vi "Main.vi"() -> ()   [LabVIEW 2017]
doc: "The myRIO Project template acquires acceleration data from the onboard accelerometer and displays the changes of acceleration values in a waveform chart."
uses:
  Motor Status Enum.ctl
  Motion Type Def.ctl
  XY Cluster.ctl
  <vilib>/addons/control/pid/pid.llb/PID Control Input Filter (DBL).vi
  <vilib>/addons/control/pid/pid.llb/PID (DBL).vi
  <vilib>/addons/control/pid/NI_PID_pid.lvlib
  <vilib>/ptbypt/NI_PtbyPt.lvlib
panel:
  out "Y Data.Path.Decel Dist":dbl
  out "X Data.Path.Decel Dist":dbl
  out "Y dist > +20":bool
  out "X dist > +20":bool
  out "Y Data.Path. Profile":T1=enum."Triangular"
  out "X Data.Path.Profile":T1=enum."Triangular"
  out "Timing":T2
  out "Y V Array":dbl[](array[numeric])
  out "X V Array":dbl[](array[numeric])
  out "Y PID":cluster{"Speed":dbl, "Speed":dbl}(graph)
  out "X PID":cluster{"Speed":dbl, "Speed":dbl}(graph)
  out "Y Data.State":T3
  out "X Data.State":T3
  out "X PID Output":dbl format="%.2f"
  out "Y PID Output":dbl format="%.2f"
  in  "Y Input":T4
  in  "Y Axis PID":cluster{"Kc":dbl, "Ti":dbl, "Td":dbl}
  in  "X Input":T4
  in  "X Axis PID":cluster{"Kc":dbl, "Ti":dbl, "Td":dbl}
  in  "stop":bool
  out "X&Y Complete":bool
  out "Y Freq":dbl(graph)
  out "X Duty%":dbl(graph)
  out "Y Acceleration":dbl[](graph)
  out "Y Displacement":dbl[](graph)
  out "X Acceleration":dbl[](graph)
  out "X Displacement":dbl[](graph)
  out "Y Velocity":cluster{"V actual":dbl[]}[](graph)
  out "X Velocity":cluster{"V actual":dbl[]}[](graph)
  out "Y Data.Motion":T5
  out "X Data.Motion":T5
  out "Y Data.Motor Params":T6
  out "X Data.Motor Params":T7
  # "X MaxV = 26.73 mm/s at 50 Hz"
  # "Y MaxV = 14.38 mm/s at 3200 µSteps/rev"
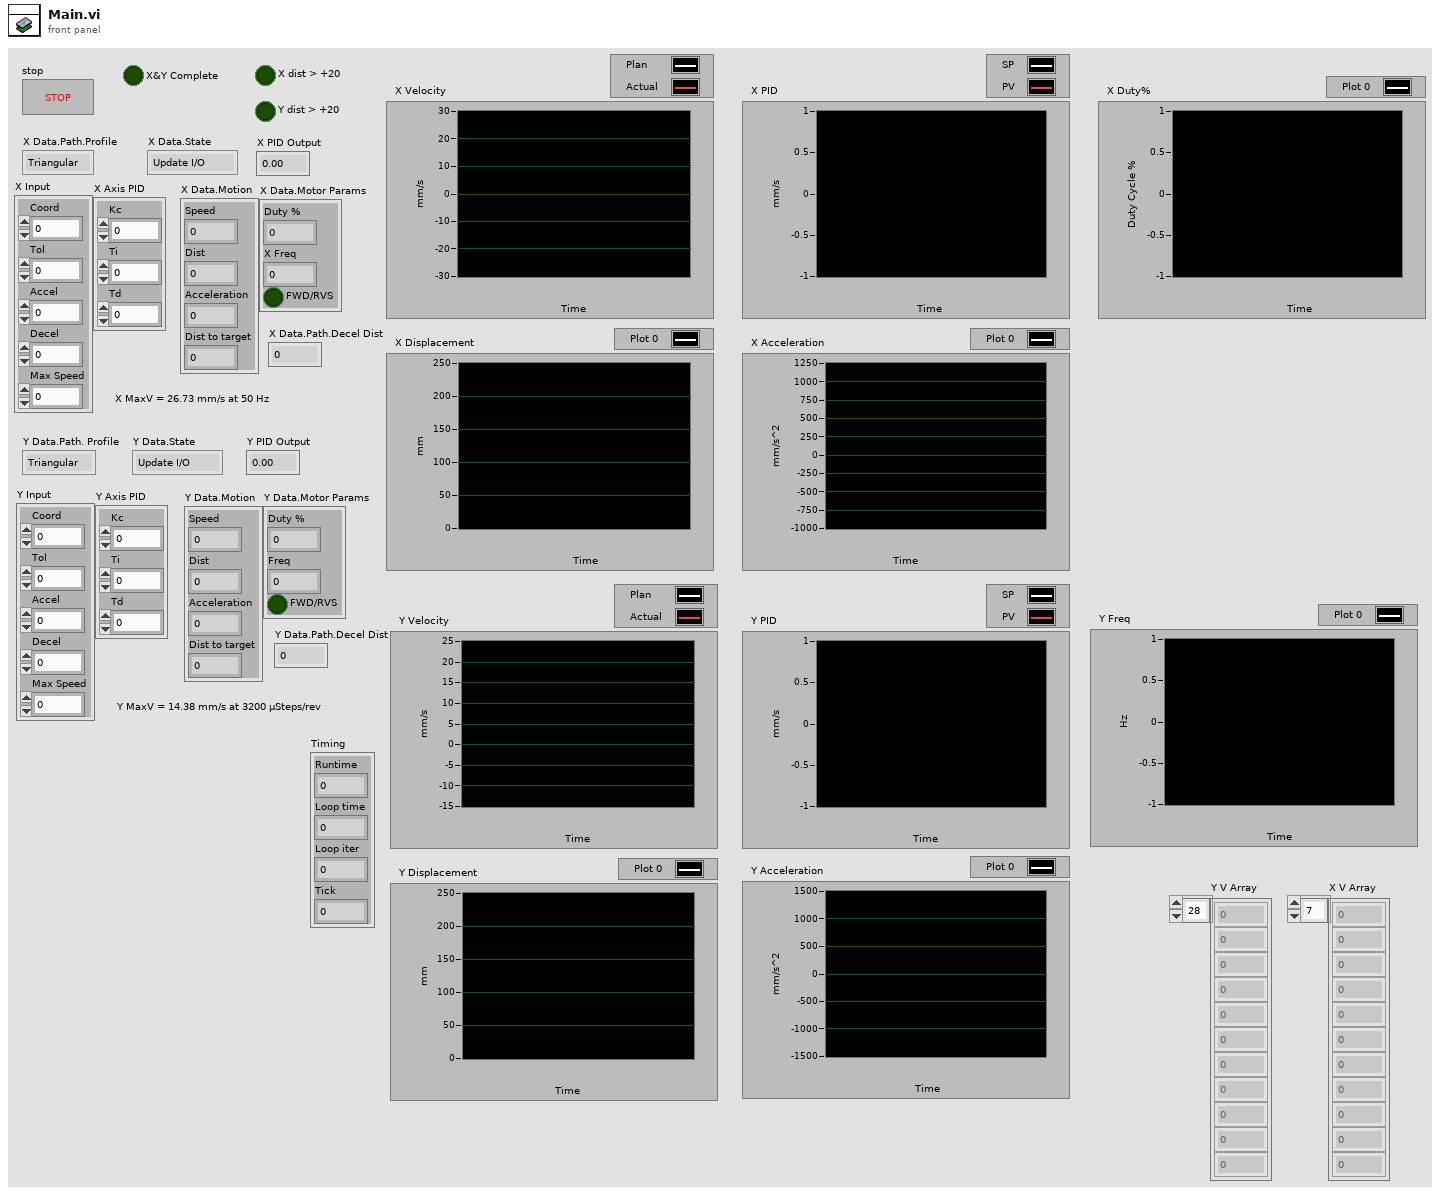
[diagram p1: front panel]
types:
  T1 = typedef "Motion Type Def.ctl" = enum16{"Trapezodial", "Triangular"}
  T2 = cluster{"Runtime":dbl, "Loop time":dbl, "Loop iter":i32, "Tick":dbl}
  T3 = typedef "Motor Status Enum.ctl" = enum16{"Update I/O", "Stop", "Steady Speed", "Accelerate", "Decelerate", "Drive Motor"}
  T4 = cluster{"Coord":dbl, "Tol":dbl, "Accel":dbl, "Decel":dbl, "Max Speed":dbl}
  T5 = cluster{"Speed":dbl, "Dist":dbl, "Acceleration":dbl, "Dist to target":dbl}
  T6 = cluster{"Duty %":dbl, "Freq":dbl, "FWD/RVS":bool}
  T7 = cluster{"Duty %":dbl, "X Freq":dbl, "FWD/RVS":bool}
  T8 = typedef "XY Cluster.ctl" = cluster{"X Data":cluster{"Complete?":bool, "Motor Params":cluster{"Duty %":dbl, "X Freq":dbl, "FWD/RVS":bool}, "SP":cluster{"Accel":dbl, "Decel":dbl, "Speed":dbl}, "State":T3, "Input":cluster{"Coord":dbl, "Tol":dbl, "Accel":dbl, "Decel":dbl, "Max Speed":dbl}, "Path":cluster{"V plan":dbl[], "V actual":dbl[], "S actual":dbl[], "a actual":dbl[], "Profile":T1, "Decel Dist":dbl, "Accel Dist":dbl, "Cruise V":dbl, "Cruise Dist":dbl}, "PID":cluster{"Kc":dbl, "Ti":dbl, "Td":dbl}, "Motion":cluster{"Speed":dbl, "Dist":dbl, "Acceleration":dbl, "Dist to target":dbl}}, "Y Data":cluster{"Complete?":bool, "Motor Params":cluster{"Duty %":dbl, "Freq":dbl, "FWD/RVS":bool}, "SP":cluster{"Y Accel":dbl, "Y Decel":dbl, "Speed":dbl}, "State":T3, "Input":cluster{"Coord":dbl, "Tol":dbl, "Accel":dbl, "Decel":dbl, "Max Speed":dbl}, "Path":cluster{"V plan":dbl[], "V actual":dbl[], "S actual":dbl[], "a actual":dbl[], " Profile":T1, "Decel Dist":dbl, "Accel Dist":dbl, "Cruise V":dbl, "Cruise Dist":dbl}, "PID":cluster{"Kc":dbl, "Ti":dbl, "Td":dbl}, "Motion":cluster{"Speed":dbl, "Dist":dbl, "Acceleration":dbl, "Dist to target":dbl}}, "Timing":cluster{"Runtime":dbl, "Loop time":dbl, "Loop iter":i32, "Tick":dbl}, "stop":bool}
  T9 = cluster{"Dist to target (mm)":dbl, "Max Speed (mm/s)":dbl, "Max Accel (mm/s^2)":dbl, "Max Decel (mm/s^2)":dbl, "Step Time (s)":dbl}
  T10 = cluster{" Distance target (mm)":dbl, "Max Accel (mm/s^2)":dbl, "Max Decel (mm/s^2)":dbl, "Velocity Limit (mm/s) ":dbl}
  T11 = cluster{"Complete?":bool, "Motor Params":cluster{"Duty %":dbl, "X Freq":dbl, "FWD/RVS":bool}, "SP":cluster{"Accel":dbl, "Decel":dbl, "Speed":dbl}, "State":T3, "Input":cluster{"Coord":dbl, "Tol":dbl, "Accel":dbl, "Decel":dbl, "Max Speed":dbl}, "Path":cluster{"V plan":dbl[], "V actual":dbl[], "S actual":dbl[], "a actual":dbl[], "Profile":T1, "Decel Dist":dbl, "Accel Dist":dbl, "Cruise V":dbl, "Cruise Dist":dbl}, "PID":cluster{"Kc":dbl, "Ti":dbl, "Td":dbl}, "Motion":cluster{"Speed":dbl, "Dist":dbl, "Acceleration":dbl, "Dist to target":dbl}}
  T12 = cluster{"Crusing Time (s)":dbl, "Decel Time (s)":dbl, "Accel Time (s)":dbl, "Total Time (s)":dbl, "Accel Distance (mm)":dbl, "Decel Distance (mm)":dbl, "Crusing Distance (mm)":dbl, "Total Dist (mm)":dbl, "Max Speed (mm/s)":dbl}
  T13 = cluster{"static gain":dbl, "lag (min)":dbl, "dead cycles":dbl, "load %":dbl, "deadband":dbl, "noise level %":dbl, "initial PV":dbl, "initial PV 2":dbl}
  T14 = cluster{"Complete?":bool, "Motor Params":cluster{"Duty %":dbl, "Freq":dbl, "FWD/RVS":bool}, "SP":cluster{"Y Accel":dbl, "Y Decel":dbl, "Speed":dbl}, "State":T3, "Input":cluster{"Coord":dbl, "Tol":dbl, "Accel":dbl, "Decel":dbl, "Max Speed":dbl}, "Path":cluster{"V plan":dbl[], "V actual":dbl[], "S actual":dbl[], "a actual":dbl[], " Profile":T1, "Decel Dist":dbl, "Accel Dist":dbl, "Cruise V":dbl, "Cruise Dist":dbl}, "PID":cluster{"Kc":dbl, "Ti":dbl, "Td":dbl}, "Motion":cluster{"Speed":dbl, "Dist":dbl, "Acceleration":dbl, "Dist to target":dbl}}
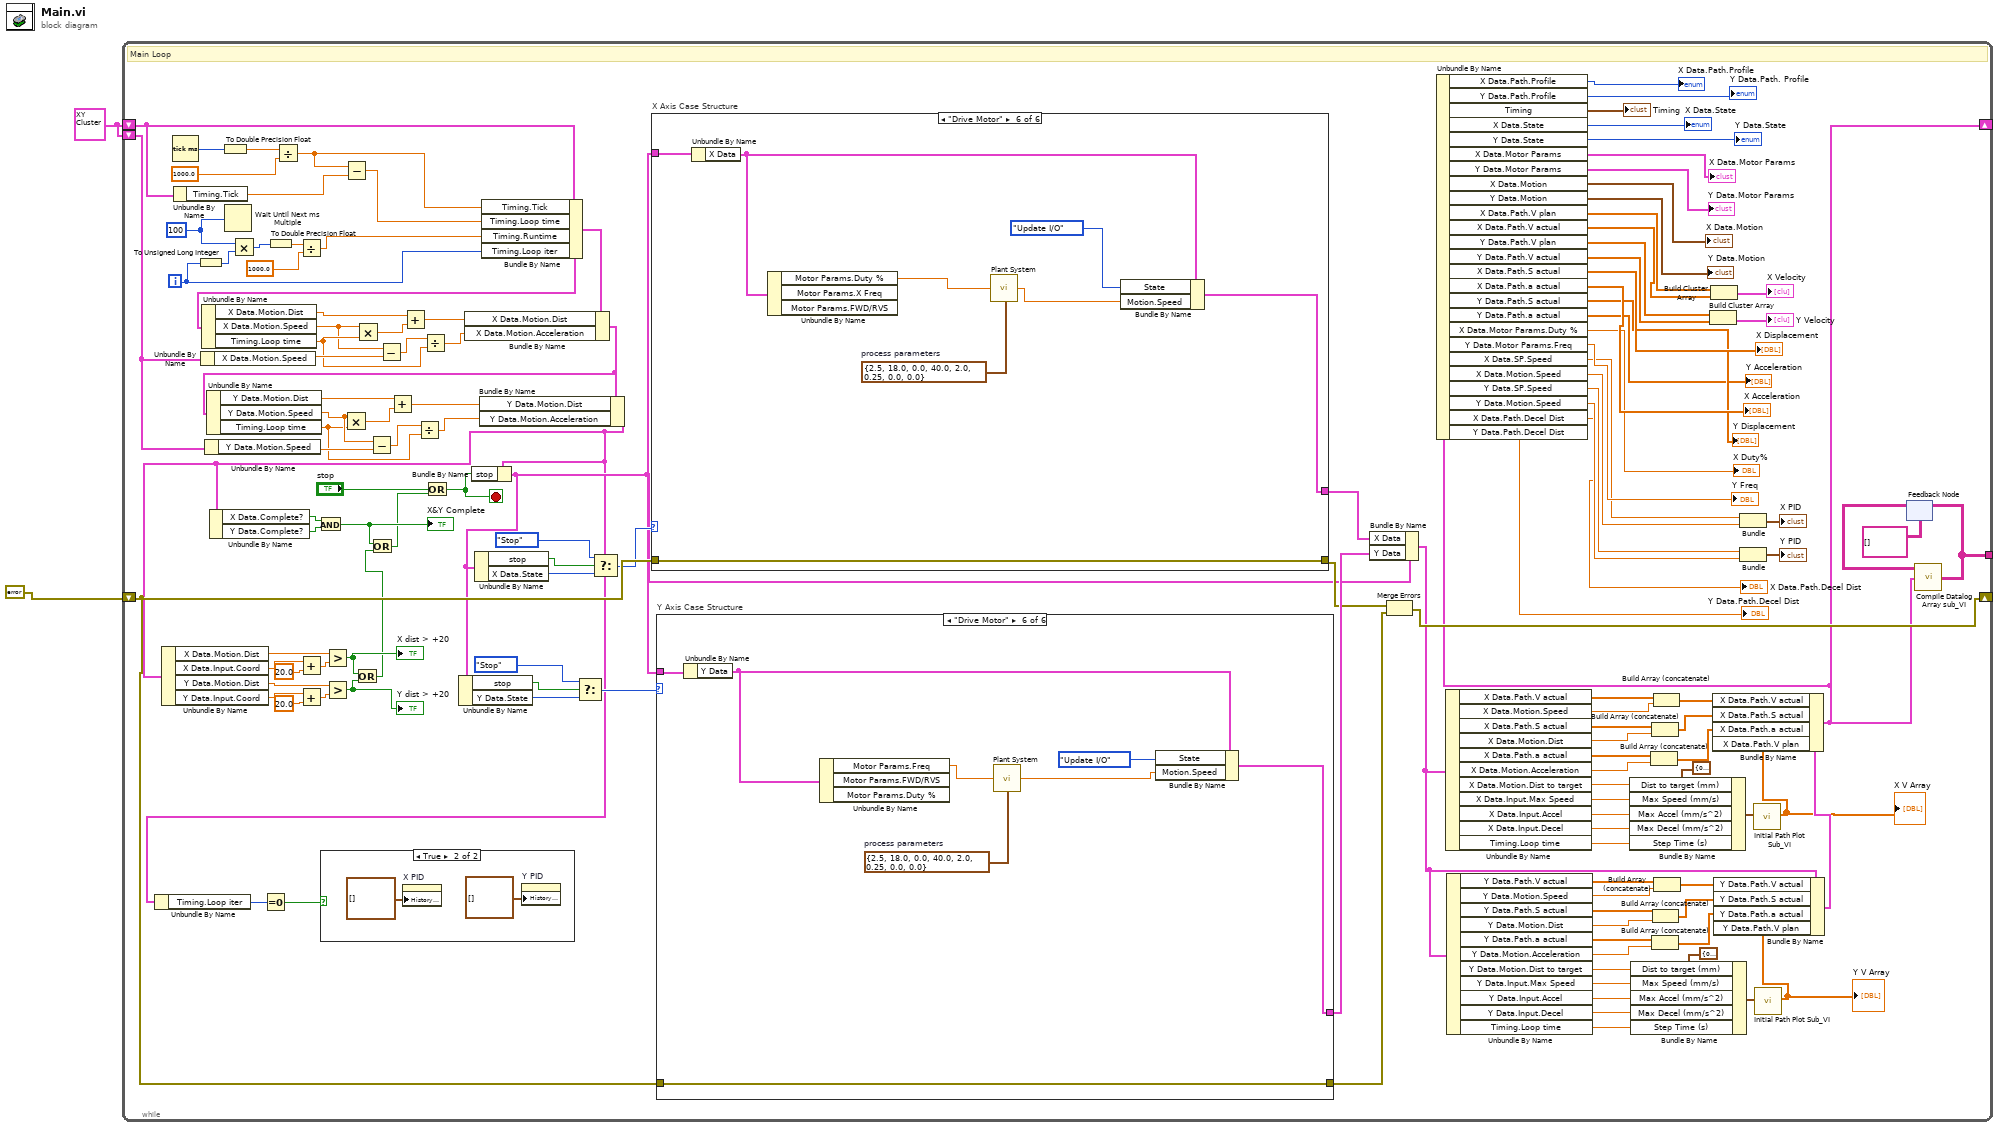
[diagram p0: block diagram]
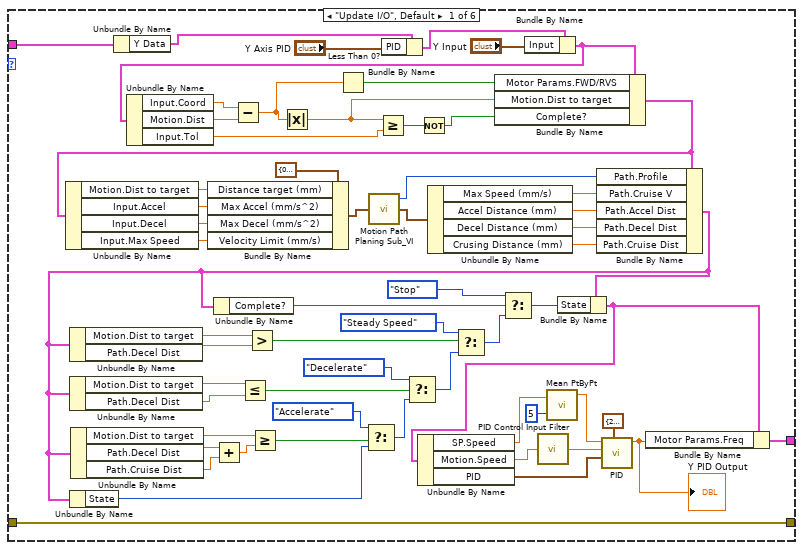
[diagram p3: hidden frame]
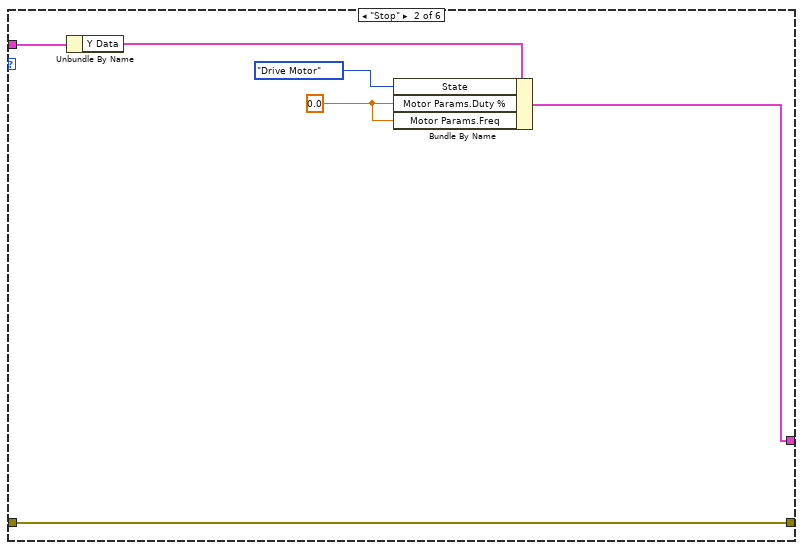
[diagram p4: hidden frame]
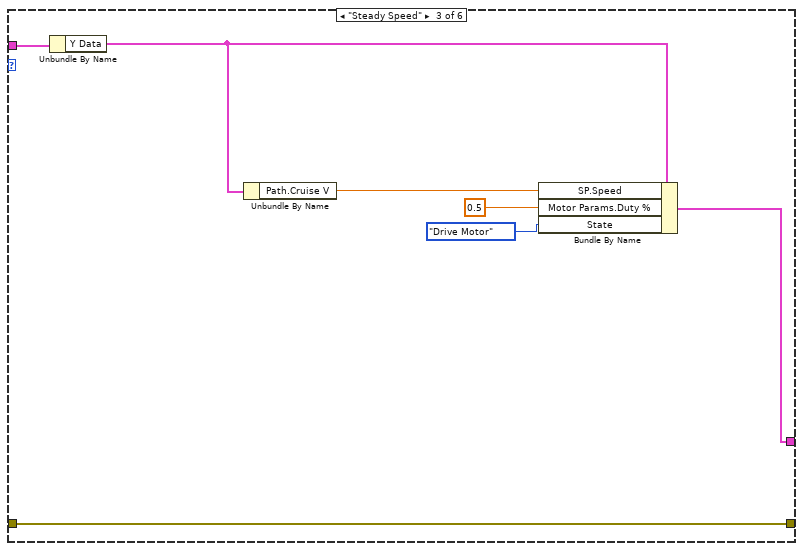
[diagram p5: hidden frame]
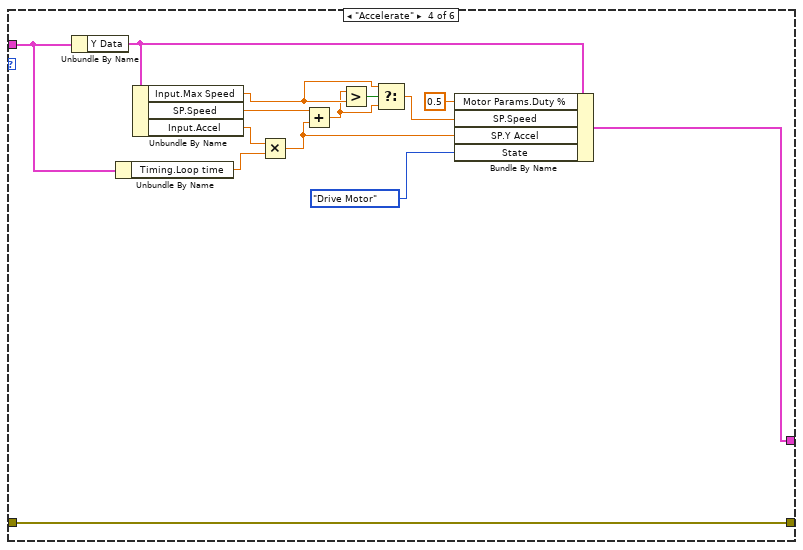
[diagram p6: hidden frame]
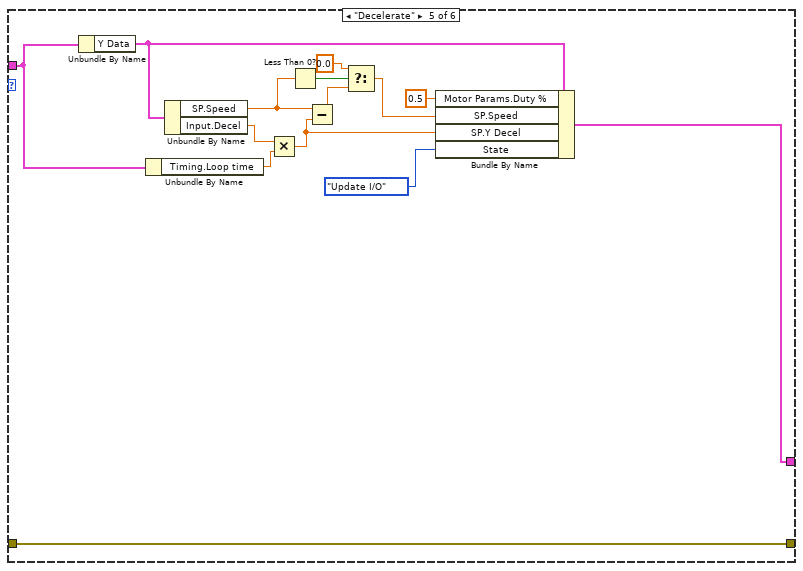
[diagram p7: hidden frame]
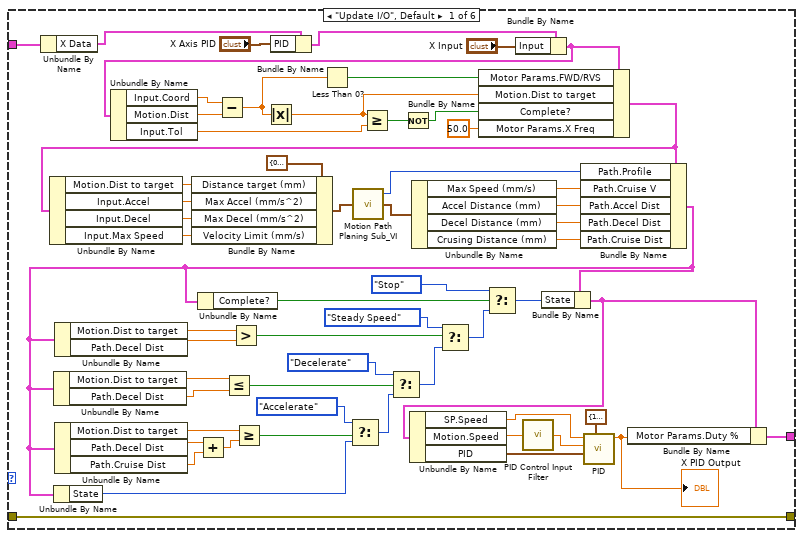
[diagram p8: hidden frame]
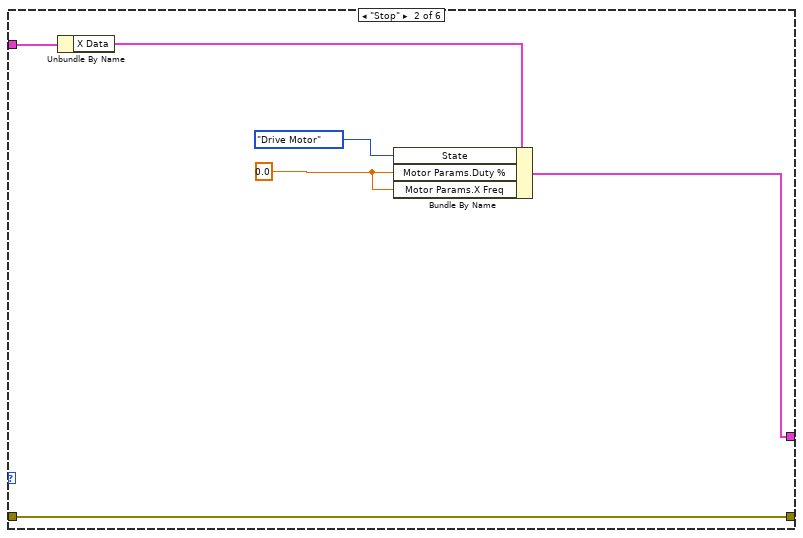
[diagram p9: hidden frame]
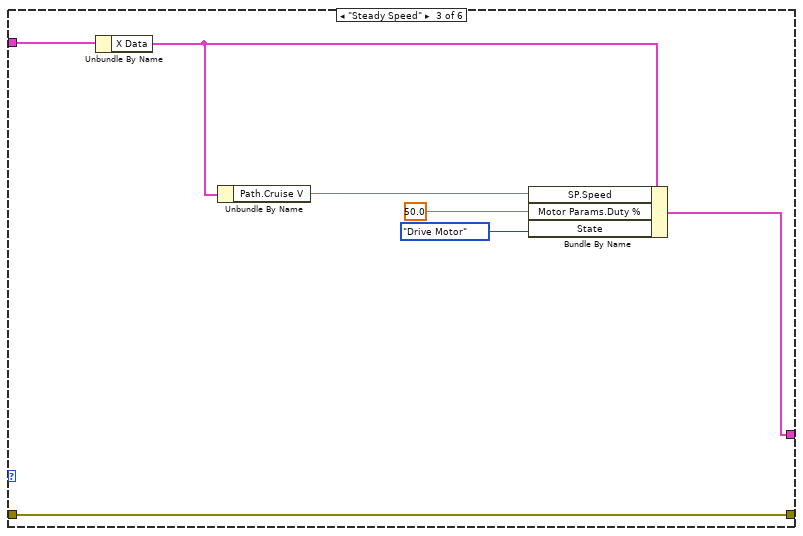
[diagram p10: hidden frame]
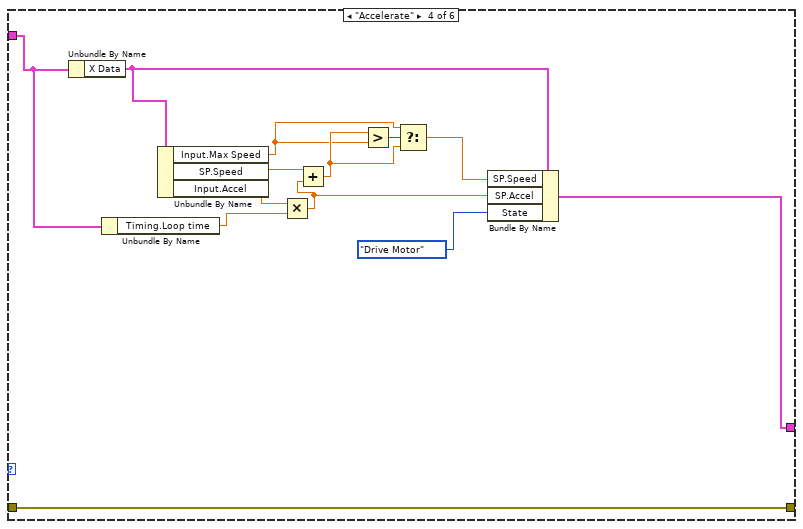
[diagram p11: hidden frame]
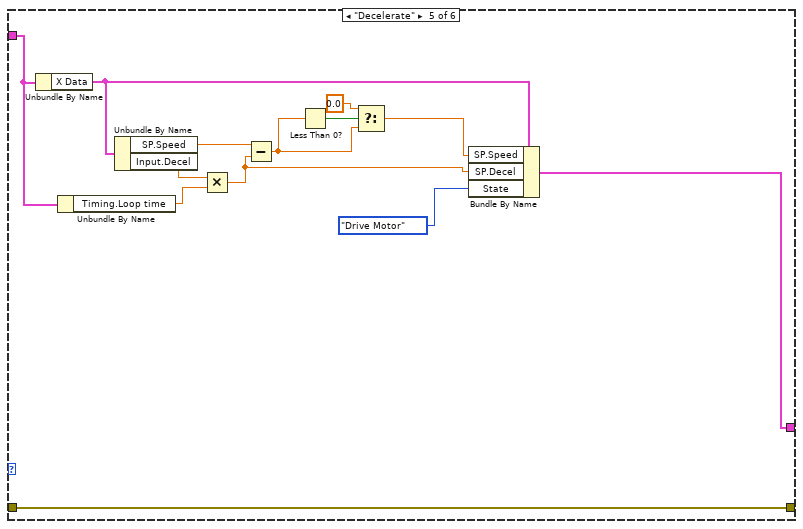
[diagram p12: hidden frame]
diagram:
  w1 = T8 {"X Data"={"Complete?"=FALSE, "Motor Params"={"Duty %"=0.0, "X Freq"=0.0, "FWD/RVS"=FALSE}, "SP"={"Accel"=0.0, "Decel"=0.0, "Speed"=0.0}, "State"=enum."Update I/O", "Input"={"Coord"=0.0, "Tol"=0.0, "Accel"=0.0, "Decel"=0.0, "Max Speed"=0.0}, "Path"={"V plan"=[], "V actual"=[], "S actual"=[], "a actual"=[], "Profile"=enum."Triangular", "Decel Dist"=0.0, "Accel Dist"=0.0, "Cruise V"=0.0, "Cruise Dist"=0.0}, "PID"={"Kc"=0.0, "Ti"=0.0, "Td"=0.0}, "Motion"={"Speed"=0.0, "Dist"=0.0, "Acceleration"=0.0, "Dist to target"=0.0}}, "Y Data"={"Complete?"=FALSE, "Motor Params"={"Duty %"=0.0, "Freq"=0.0, "FWD/RVS"=FALSE}, "SP"={"Y Accel"=0.0, "Y Decel"=0.0, "Speed"=0.0}, "State"=enum."Update I/O", "Input"={"Coord"=0.0, "Tol"=0.0, "Accel"=0.0, "Decel"=0.0, "Max Speed"=0.0}, "Path"={"V plan"=[], "V actual"=[], "S actual"=[], "a actual"=[], " Profile"=enum."Triangular", "Decel Dist"=0.0, "Accel Dist"=0.0, "Cruise V"=0.0, "Cruise Dist"=0.0}, "PID"={"Kc"=0.0, "Ti"=0.0, "Td"=0.0}, "Motion"={"Speed"=0.0, "Dist"=0.0, "Acceleration"=0.0, "Dist to target"=0.0}}, "Timing"={"Runtime"=0.0, "Loop time"=0.0, "Loop iter"=0, "Tick"=0.0}, "stop"=FALSE} ("XY Cluster 2")
  n1 = while {
    shift-right: [w125] -> _
    shift-left: errorcluster {"status"=FALSE, "code"=0, "source"=""} ("error in (no error)") -> [w127]
    shift-right: [w40] -> _
    shift-left: w1 -> [w54]
    tunnel: [w122] -> _
    shift-left: w1 -> [w9]
    i -> [w137]
    stop <- w20 stop-if-true
    w136 = u32 100 ("millisecond multiple")
    # "Main Loop"
    n2 = Tick Count (ms)() -> (millisecond timer value=w130:u32)
    n3 = Unbundle By Name(w54) -> ("Timing.Tick"=w53:dbl)
    n4 = To Unsigned Long Integer(number=w137) -> (unsigned 32bit integer=w135:u32)
    n5 = Unbundle By Name(w9) -> ("X Data.Motion.Speed"=w13:dbl)
    n6 = Unbundle By Name(w9) -> ("Y Data.Motion.Speed"=w6:dbl)
    n7 = To Double Precision Float(number=w130) -> (double precision float=w55:dbl)
    n8 = Wait Until Next ms Multiple(millisecond multiple=w136) -> ()  [unwired: 1 out]
    n9 = Multiply(x=w136, y=w135) -> (x*y=w134:u32)
    n10 = To Double Precision Float(number=w134) -> (double precision float=w132:dbl)
    n11 = Divide(x=w55, y=1000.0) -> (x/y=w52:dbl)
    n12 = Divide(x=w132, y=1000.0) -> (x/y=w131:dbl)
    n13 = Subtract(x=w52, y=w53) -> (x-y=w51:dbl)
    n14 = Bundle By Name(cluster=w54, "Timing.Tick"=w52, "Timing.Loop time"=w51, "Timing.Runtime"=w131, "Timing.Loop iter"=w137) -> (w138:T8)
    n15 = Unbundle By Name(w138) -> ("X Data.Motion.Dist"=w19:dbl, "X Data.Motion.Speed"=w8:dbl, "Timing.Loop time"=w11:dbl)
    n16 = Multiply(x=w8, y=w11) -> (x*y=w14:dbl)
    n17 = Subtract(x=w8, y=w13) -> (x-y=w12:dbl)
    n18 = Add(x=w19, y=w14) -> (x+y=w18:dbl)
    n19 = Divide(x=w12, y=w11) -> (x/y=w10:dbl)
    n20 = Bundle By Name(cluster=w138, "X Data.Motion.Dist"=w18, "X Data.Motion.Acceleration"=w10) -> (w128:T8)
    n21 = Unbundle By Name(w128) -> ("Y Data.Motion.Dist"=w17:dbl, "Y Data.Motion.Speed"=w7:dbl, "Timing.Loop time"=w4:dbl)
    n22 = Multiply(x=w7, y=w4) -> (x*y=w16:dbl)
    n23 = Subtract(x=w7, y=w6) -> (x-y=w5:dbl)
    n24 = Add(x=w17, y=w16) -> (x+y=w15:dbl)
    n25 = Divide(x=w5, y=w4) -> (x/y=w3:dbl)
    n26 = Bundle By Name(cluster=w128, "Y Data.Motion.Dist"=w15, "Y Data.Motion.Acceleration"=w3) -> (w25:T8)
    n27 = Unbundle By Name(w25) -> ("Timing.Loop iter"=w23:i32)
    n28 = Unbundle By Name(w25) -> ("X Data.Motion.Dist"=w39:dbl, "X Data.Input.Coord"=w32:dbl, "Y Data.Motion.Dist"=w37:dbl, "Y Data.Input.Coord"=w29:dbl)
    n29 = Unbundle By Name(w25) -> ("X Data.Complete?"=w107:bool, "Y Data.Complete?"=w106:bool)
    n30 = Equal To 0?(x=w23) -> (x = 0?=w24:bool)
    n31 = Add(x=w32, y=20.0) -> (x+y=w31:dbl)
    n32 = Add(x=w29, y=20.0) -> (x+y=w28:dbl)
    n33 = And(x=w107, y=w106) -> (x .and. y?=w35:bool)
    "X&Y Complete" <- w35
    n34 = case shown="True" w24 {
      frame False {
      }
      frame True {
        n35 = property on="X PID" class="WFChart (strict)"("History Data"=cluster{"Speed":dbl, "Speed":dbl}[] []) -> ()  [unwired: 2 in, 2 out]
        n36 = property on="Y PID" class="WFChart (strict)"("History Data"=cluster{"Speed":dbl, "Speed":dbl}[] []) -> ()  [unwired: 2 in, 2 out]
      }
    }
    n37 = Greater?(x=w39, y=w31) -> (0:w38:bool)
    "X dist > +20" <- w38
    n38 = Greater?(x=w37, y=w28) -> (0:w34:bool)
    "Y dist > +20" <- w34
    n39 = Or(x=w38, y=w34) -> (x .or. y?=w36:bool)
    n40 = Or(x=w35, y=w36) -> (x .or. y?=w21:bool)
    n41 = Or(x="stop", y=w21) -> (x .or. y?=w20:bool)
    n42 = Bundle By Name(cluster=w25, "stop"=w20) -> (w47:T8)
    n43 = Unbundle By Name(w47) -> ("stop"=w110:bool, "Y Data.State"=w111:T3)
    n44 = Unbundle By Name(w47) -> ("stop"=w114:bool, "X Data.State"=w115:T3)
    n45 = Select(t=Motor_Status_Enum."Stop", s=w110, f=w111) -> (s? t:f=w108:T3)
    n46 = Select(t=Motor_Status_Enum."Stop", s=w114, f=w115) -> (s? t:f=w112:T3)
    n47 = case "X Axis Case Structure" shown="\"Drive Motor\"" w112 {
      tunnel: [w278 w315 w320 w334 w342 w354] -> w139
      tunnel: w127 -> [w299 w310 w318 w332 w341 w352]
      tunnel: [w299 w310 w318 w332 w341 w352] -> w124
      tunnel: w47 -> [w279 w312 w321 w333 w344 w356]
      frame "Update I/O", Default {
        n48 = Unbundle By Name(w279) -> ("X Data"=w258:T11)
        n49 = Bundle By Name(cluster=w258, "PID"="X Axis PID") -> (w261:T11)
        n50 = Bundle By Name(cluster=w261, "Input"="X Input") -> (w257:T11)
        n51 = Unbundle By Name(w257) -> ("Input.Coord"=w309:dbl, "Motion.Dist"=w304:dbl, "Input.Tol"=w308:dbl)
        n52 = Subtract(x=w309, y=w304) -> (x-y=w305:dbl)
        n53 = Absolute Value(x=w305) -> (abs(x)=w276:dbl)
        n54 = Less Than 0?(x=w305) -> (x < 0?=w277:bool)
        n55 = Greater Or Equal?(x=w276, y=w308) -> (x >= y?=w307:bool)
        n56 = Not(x=w307) -> (.not. x?=w306:bool)
        n57 = Bundle By Name(cluster=w257, "Motor Params.FWD/RVS"=w277, "Motion.Dist to target"=w276, "Complete?"=w306, "Motor Params.X Freq"=50.0) -> (w274:T11)
        n58 = Unbundle By Name(w274) -> ("Motion.Dist to target"=w275:dbl, "Input.Accel"=w296:dbl, "Input.Decel"=w295:dbl, "Input.Max Speed"=w297:dbl)
        n59 = Bundle By Name(cluster=T10 {" Distance target (mm)"=0.0, "Max Accel (mm/s^2)"=0.0, "Max Decel (mm/s^2)"=0.0, "Velocity Limit (mm/s) "=0.0} ("Motion Planning Inputs"), "Distance target (mm)"=w275, "Max Accel (mm/s^2)"=w296, "Max Decel (mm/s^2)"=w295, "Velocity Limit (mm/s)"=w297) -> (w253:T10)
        n60 = call "Motion Path Planing Sub_VI.vi"("Motion Planning Inputs"=w253) -> ("Motion Profile"=w252:T1, "Motion Planning Outputs"=w251:T12)  [unwired: 5 in]
        n61 = Unbundle By Name(w251) -> ("Max Speed (mm/s)"=w298:dbl, "Accel Distance (mm)"=w293:dbl, "Decel Distance (mm)"=w292:dbl, "Crusing Distance (mm)"=w273:dbl)
        n62 = Bundle By Name(cluster=w274, "Path.Profile"=w252, "Path.Cruise V"=w298, "Path.Accel Dist"=w293, "Path.Decel Dist"=w292, "Path.Cruise Dist"=w273) -> (w268:T11)
        n63 = Unbundle By Name(w268) -> ("Motion.Dist to target"=w270:dbl, "Path.Decel Dist"=w269:dbl)
        n64 = Unbundle By Name(w268) -> ("State"=w290:T3)
        n65 = Unbundle By Name(w268) -> ("Motion.Dist to target"=w272:dbl, "Path.Decel Dist"=w271:dbl)
        n66 = Unbundle By Name(w268) -> ("Motion.Dist to target"=w264:dbl, "Path.Decel Dist"=w267:dbl, "Path.Cruise Dist"=w266:dbl)
        n67 = Unbundle By Name(w268) -> ("Complete?"=w282:bool)
        n68 = Add(x=w267, y=w266) -> (x+y=w265:dbl)
        n69 = Less Or Equal?(x=w270, y=w269) -> (x <= y?=w289:bool)
        n70 = Greater?(x=w272, y=w271) -> (0:w285:bool)
        n71 = Greater Or Equal?(x=w264, y=w265) -> (x >= y?=w263:bool)
        n72 = Select(t=Motor_Status_Enum."Accelerate" ("State"), s=w263, f=w290) -> (s? t:f=w288:T3)
        n73 = Select(t=Motor_Status_Enum."Decelerate" ("State"), s=w289, f=w288) -> (s? t:f=w284:T3)
        n74 = Select(t=Motor_Status_Enum."Steady Speed" ("State"), s=w285, f=w284) -> (s? t:f=w283:T3)
        n75 = Select(t=Motor_Status_Enum."Stop" ("State"), s=w282, f=w283) -> (s? t:f=w280:T3)
        n76 = Bundle By Name(cluster=w268, "State"=w280) -> (w259:T11)
        n77 = Unbundle By Name(w259) -> ("SP.Speed"=w294:dbl, "Motion.Speed"=w302:dbl, "PID"=w301:cluster{"Kc":dbl, "Ti":dbl, "Td":dbl})
        n78 = call-poly <vilib>:"PID Control Input Filter.vi"("input"=w302) -> ("output"=w303:dbl)  [unwired: 4 in]
        n79 = call-poly <vilib>:"PID.vi"("output range"=cluster{"output high":dbl, "output low":dbl} {"output high"=100.0, "output low"=0.0}, "PID gains"=w301, "process variable"=w303, "setpoint"=w294) -> ("output"=w256:dbl)  [unwired: 6 in, 1 out]
        "X PID Output" <- w256
        n80 = Bundle By Name(cluster=w259, "Motor Params.Duty %"=w256) -> (w278:T11)
      }
      frame "Stop" {
        w314 = 0.0
        n81 = Unbundle By Name(w312) -> ("X Data"=w311:T11)
        n82 = Bundle By Name(cluster=w311, "State"=Motor_Status_Enum."Drive Motor", "Motor Params.Duty %"=w314, "Motor Params.X Freq"=w314) -> (w315:T11)
      }
      frame "Steady Speed" {
        n83 = Unbundle By Name(w321) -> ("X Data"=w317:T11)
        n84 = Unbundle By Name(w317) -> ("Path.Cruise V"=w316:dbl)
        n85 = Bundle By Name(cluster=w317, "SP.Speed"=w316, "Motor Params.Duty %"=50.0, "State"=Motor_Status_Enum."Drive Motor") -> (w320:T11)
      }
      frame "Accelerate" {
        n86 = Unbundle By Name(w333) -> ("X Data"=w335:T11)
        n87 = Unbundle By Name(w333) -> ("Timing.Loop time"=w331:dbl)
        n88 = Unbundle By Name(w335) -> ("Input.Max Speed"=w323:dbl, "SP.Speed"=w329:dbl, "Input.Accel"=w328:dbl)
        n89 = Multiply(x=w328, y=w331) -> (x*y=w327:dbl)
        n90 = Add(x=w329, y=w327) -> (x+y=w324:dbl)
        n91 = Greater?(x=w324, y=w323) -> (0:w326:bool)
        n92 = Select(t=w323, s=w326, f=w324) -> (s? t:f=w325:dbl)
        n93 = Bundle By Name(cluster=w335, "SP.Speed"=w325, "SP.Accel"=w327, "State"=Motor_Status_Enum."Drive Motor") -> (w334:T11)
      }
      frame "Decelerate" {
        n94 = Unbundle By Name(w344) -> ("X Data"=w343:T11)
        n95 = Unbundle By Name(w344) -> ("Timing.Loop time"=w348:dbl)
        n96 = Unbundle By Name(w343) -> ("SP.Speed"=w346:dbl, "Input.Decel"=w345:dbl)
        n97 = Multiply(x=w345, y=w348) -> (x*y=w340:dbl)
        n98 = Subtract(x=w346, y=w340) -> (x-y=w336:dbl)
        n99 = Less Than 0?(x=w336) -> (x < 0?=w339:bool)
        n100 = Select(t=0.0, s=w339, f=w336) -> (s? t:f=w338:dbl)
        n101 = Bundle By Name(cluster=w343, "SP.Speed"=w338, "SP.Decel"=w340, "State"=Motor_Status_Enum."Drive Motor") -> (w342:T11)
      }
      frame "Drive Motor" {
        w350 = T13 {"static gain"=2.5, "lag (min)"=18.0, "dead cycles"=0.0, "load %"=40.0, "deadband"=2.0, "noise level %"=0.25, "initial PV"=0.0, "initial PV 2"=0.0}  # process parameters
        n102 = Unbundle By Name(w356) -> ("X Data"=w355:T11)
        n103 = Unbundle By Name(w355) -> ("Motor Params.Duty %"=w349:dbl)  [unwired: 2 out]
        n104 = call "Plant System.vi"("Plant Input"=w349, "process parameters"=w350) -> ("Plant Output"=w351:dbl)  [unwired: 13 in]
        n105 = Bundle By Name(cluster=w355, "State"=Motor_Status_Enum."Update I/O", "Motion.Speed"=w351) -> (w354:T11)
      }
    }
    n106 = case "Y Axis Case Structure" shown="\"Drive Motor\"" w108 {
      tunnel: [w155 w207 w212 w227 w237 w248] -> w126
      tunnel: w127 -> [w201 w202 w211 w225 w236 w243]
      tunnel: [w201 w202 w211 w225 w236 w243] -> w123
      tunnel: w47 -> [w200 w204 w213 w226 w239 w250]
      frame "Update I/O", Default {
        n107 = Unbundle By Name(w200) -> ("Y Data"=w151:T14)
        n108 = Bundle By Name(cluster=w151, "PID"="Y Axis PID") -> (w153:T14)
        n109 = Bundle By Name(cluster=w153, "Input"="Y Input") -> (w150:T14)
        n110 = Unbundle By Name(w150) -> ("Input.Coord"=w199:dbl, "Motion.Dist"=w195:dbl, "Input.Tol"=w198:dbl)
        n111 = Subtract(x=w199, y=w195) -> (x-y=w158:dbl)
        n112 = Absolute Value(x=w158) -> (abs(x)=w171:dbl)
        n113 = Less Than 0?(x=w158) -> (x < 0?=w157:bool)
        n114 = Greater Or Equal?(x=w171, y=w198) -> (x >= y?=w197:bool)
        n115 = Not(x=w197) -> (.not. x?=w196:bool)
        n116 = Bundle By Name(cluster=w150, "Motor Params.FWD/RVS"=w157, "Motion.Dist to target"=w171, "Complete?"=w196) -> (w169:T14)
        n117 = Unbundle By Name(w169) -> ("Motion.Dist to target"=w170:dbl, "Input.Accel"=w187:dbl, "Input.Decel"=w186:dbl, "Input.Max Speed"=w188:dbl)
        n118 = Bundle By Name(cluster=T10 {" Distance target (mm)"=0.0, "Max Accel (mm/s^2)"=0.0, "Max Decel (mm/s^2)"=0.0, "Velocity Limit (mm/s) "=0.0} ("Motion Planning Inputs"), "Distance target (mm)"=w170, "Max Accel (mm/s^2)"=w187, "Max Decel (mm/s^2)"=w186, "Velocity Limit (mm/s)"=w188) -> (w144:T10)
        n119 = call "Motion Path Planing Sub_VI.vi"("Motion Planning Inputs"=w144) -> ("Motion Profile"=w143:T1, "Motion Planning Outputs"=w142:T12)  [unwired: 5 in]
        n120 = Unbundle By Name(w142) -> ("Max Speed (mm/s)"=w189:dbl, "Accel Distance (mm)"=w185:dbl, "Decel Distance (mm)"=w184:dbl, "Crusing Distance (mm)"=w168:dbl)
        n121 = Bundle By Name(cluster=w169, "Path.Profile"=w143, "Path.Cruise V"=w189, "Path.Accel Dist"=w185, "Path.Decel Dist"=w184, "Path.Cruise Dist"=w168) -> (w156:T14)
        n122 = Unbundle By Name(w156) -> ("Motion.Dist to target"=w167:dbl, "Path.Decel Dist"=w166:dbl)
        n123 = Unbundle By Name(w156) -> ("Motion.Dist to target"=w165:dbl, "Path.Decel Dist"=w164:dbl)
        n124 = Unbundle By Name(w156) -> ("State"=w182:T3)
        n125 = Unbundle By Name(w156) -> ("Motion.Dist to target"=w160:dbl, "Path.Decel Dist"=w163:dbl, "Path.Cruise Dist"=w162:dbl)
        n126 = Unbundle By Name(w156) -> ("Complete?"=w174:bool)
        n127 = Add(x=w163, y=w162) -> (x+y=w161:dbl)
        n128 = Less Or Equal?(x=w165, y=w164) -> (x <= y?=w181:bool)
        n129 = Greater?(x=w167, y=w166) -> (0:w177:bool)
        n130 = Greater Or Equal?(x=w160, y=w161) -> (x >= y?=w159:bool)
        n131 = Select(t=Motor_Status_Enum."Accelerate" ("State"), s=w159, f=w182) -> (s? t:f=w180:T3)
        n132 = Select(t=Motor_Status_Enum."Decelerate" ("State"), s=w181, f=w180) -> (s? t:f=w176:T3)
        n133 = Select(t=Motor_Status_Enum."Steady Speed" ("State"), s=w177, f=w176) -> (s? t:f=w175:T3)
        n134 = Select(t=Motor_Status_Enum."Stop" ("State"), s=w174, f=w175) -> (s? t:f=w172:T3)
        n135 = Bundle By Name(cluster=w156, "State"=w172) -> (w149:T14)
        n136 = Unbundle By Name(w149) -> ("SP.Speed"=w147:dbl, "Motion.Speed"=w193:dbl, "PID"=w192:cluster{"Kc":dbl, "Ti":dbl, "Td":dbl})
        n137 = call-poly <vilib>:"PID Control Input Filter.vi"("input"=w193) -> ("output"=w194:dbl)  [unwired: 4 in]
        n138 = call <vilib>:"Mean PtByPt.vi"("x"=w147, "sample length"=5) -> ("mean"=w148:dbl)  [unwired: 2 in, 1 out]
        n139 = call-poly <vilib>:"PID.vi"("output range"=cluster{"output high":dbl, "output low":dbl} {"output high"=23000.0, "output low"=0.0}, "PID gains"=w192, "process variable"=w194, "setpoint"=w148) -> ("output"=w190:dbl)  [unwired: 6 in, 1 out]
        "Y PID Output" <- w190
        n140 = Bundle By Name(cluster=w149, "Motor Params.Freq"=w190) -> (w155:T14)
      }
      frame "Stop" {
        w206 = 0.0
        n141 = Unbundle By Name(w204) -> ("Y Data"=w203:T14)
        n142 = Bundle By Name(cluster=w203, "State"=Motor_Status_Enum."Drive Motor", "Motor Params.Duty %"=w206, "Motor Params.Freq"=w206) -> (w207:T14)
      }
      frame "Steady Speed" {
        n143 = Unbundle By Name(w213) -> ("Y Data"=w209:T14)
        n144 = Unbundle By Name(w209) -> ("Path.Cruise V"=w208:dbl)
        n145 = Bundle By Name(cluster=w209, "SP.Speed"=w208, "Motor Params.Duty %"=0.5, "State"=Motor_Status_Enum."Drive Motor") -> (w212:T14)
      }
      frame "Accelerate" {
        n146 = Unbundle By Name(w226) -> ("Y Data"=w228:T14)
        n147 = Unbundle By Name(w226) -> ("Timing.Loop time"=w224:dbl)
        n148 = Unbundle By Name(w228) -> ("Input.Max Speed"=w216:dbl, "SP.Speed"=w222:dbl, "Input.Accel"=w221:dbl)
        n149 = Multiply(x=w221, y=w224) -> (x*y=w220:dbl)
        n150 = Add(x=w222, y=w220) -> (x+y=w215:dbl)
        n151 = Greater?(x=w215, y=w216) -> (0:w218:bool)
        n152 = Select(t=w216, s=w218, f=w215) -> (s? t:f=w217:dbl)
        n153 = Bundle By Name(cluster=w228, "Motor Params.Duty %"=0.5, "SP.Speed"=w217, "SP.Y Accel"=w220, "State"=Motor_Status_Enum."Drive Motor") -> (w227:T14)
      }
      frame "Decelerate" {
        n154 = Unbundle By Name(w239) -> ("Y Data"=w238:T14)
        n155 = Unbundle By Name(w239) -> ("Timing.Loop time"=w242:dbl)
        n156 = Unbundle By Name(w238) -> ("SP.Speed"=w232:dbl, "Input.Decel"=w240:dbl)
        n157 = Multiply(x=w240, y=w242) -> (x*y=w235:dbl)
        n158 = Less Than 0?(x=w232) -> (x < 0?=w233:bool)
        n159 = Subtract(x=w232, y=w235) -> (x-y=w229:dbl)
        n160 = Select(t=0.0, s=w233, f=w229) -> (s? t:f=w231:dbl)
        n161 = Bundle By Name(cluster=w238, "Motor Params.Duty %"=0.5, "SP.Speed"=w231, "SP.Y Decel"=w235, "State"=Motor_Status_Enum."Update I/O") -> (w237:T14)
      }
      frame "Drive Motor" {
        w245 = T13 {"static gain"=2.5, "lag (min)"=18.0, "dead cycles"=0.0, "load %"=40.0, "deadband"=2.0, "noise level %"=0.25, "initial PV"=0.0, "initial PV 2"=0.0}  # process parameters
        n162 = Unbundle By Name(w250) -> ("Y Data"=w249:T14)
        n163 = Unbundle By Name(w249) -> ("Motor Params.Freq"=w246:dbl)  [unwired: 2 out]
        n164 = call "Plant System.vi"("Plant Input"=w246, "process parameters"=w245) -> ("Plant Output"=w244:dbl)  [unwired: 13 in]
        n165 = Bundle By Name(cluster=w249, "State"=Motor_Status_Enum."Update I/O", "Motion.Speed"=w244) -> (w248:T14)
      }
    }
    n166 = Bundle By Name(cluster=w47, "X Data"=w139, "Y Data"=w126) -> (w67:T8)
    n167 = Merge Errors(w124, w123) -> (w125:errorcluster)
    n168 = Unbundle By Name(w67) -> ("X Data.Path.V actual"=w99:dbl[], "X Data.Motion.Speed"=w98:dbl, "X Data.Path.S actual"=w95:dbl[], "X Data.Motion.Dist"=w94:dbl, "X Data.Path.a actual"=w93:dbl[], "X Data.Motion.Acceleration"=w92:dbl, "X Data.Motion.Dist to target"=w88:dbl, "X Data.Input.Max Speed"=w87:dbl, "X Data.Input.Accel"=w86:dbl, "X Data.Input.Decel"=w85:dbl, "Timing.Loop time"=w84:dbl)
    n169 = Unbundle By Name(w67) -> ("Y Data.Path.V actual"=w83:dbl[], "Y Data.Motion.Speed"=w82:dbl, "Y Data.Path.S actual"=w79:dbl[], "Y Data.Motion.Dist"=w78:dbl, "Y Data.Path.a actual"=w77:dbl[], "Y Data.Motion.Acceleration"=w76:dbl, "Y Data.Motion.Dist to target"=w72:dbl, "Y Data.Input.Max Speed"=w71:dbl, "Y Data.Input.Accel"=w70:dbl, "Y Data.Input.Decel"=w69:dbl, "Timing.Loop time"=w68:dbl)
    n170 = Bundle By Name(cluster=T9 {"Dist to target (mm)"=0.0, "Max Speed (mm/s)"=0.0, "Max Accel (mm/s^2)"=0.0, "Max Decel (mm/s^2)"=0.0, "Step Time (s)"=0.0} ("Motion Inputs"), "Dist to target (mm)"=w88, "Max Speed (mm/s)"=w87, "Max Accel (mm/s^2)"=w86, "Max Decel (mm/s^2)"=w85, "Step Time (s)"=w84) -> (w90:T9)
    n171 = Bundle By Name(cluster=T9 {"Dist to target (mm)"=0.0, "Max Speed (mm/s)"=0.0, "Max Accel (mm/s^2)"=0.0, "Max Decel (mm/s^2)"=0.0, "Step Time (s)"=0.0} ("Motion Inputs"), "Dist to target (mm)"=w72, "Max Speed (mm/s)"=w71, "Max Accel (mm/s^2)"=w70, "Max Decel (mm/s^2)"=w69, "Step Time (s)"=w68) -> (w74:T9)
    n172 = Build Array (concatenate)(w93, w92) -> (w91:dbl[])
    n173 = Build Array (concatenate)(w95, w94) -> (w96:dbl[])
    n174 = Build Array (concatenate)(w77, w76) -> (w75:dbl[])
    n175 = Build Array (concatenate)(w79, w78) -> (w80:dbl[])
    n176 = Build Array (concatenate)(w99, w98) -> (w97:dbl[])
    n177 = Build Array (concatenate)(w83, w82) -> (w81:dbl[])
    n178 = call "Initial Path Plot Sub_VI.vi"("Motion Inputs"=w90) -> ("Velocity Array"=w56:dbl[])  [unwired: 7 in, 3 out]
    "X V Array" <- w56
    n179 = call "Initial Path Plot Sub_VI.vi"("Motion Inputs"=w74) -> ("Velocity Array"=w57:dbl[])  [unwired: 7 in, 3 out]
    "Y V Array" <- w57
    n180 = Bundle By Name(cluster=w67, "Y Data.Path.V actual"=w81, "Y Data.Path.S actual"=w80, "Y Data.Path.a actual"=w75, "Y Data.Path.V plan"=w57) -> (w66:T8)
    n181 = Bundle By Name(cluster=w66, "X Data.Path.V actual"=w97, "X Data.Path.S actual"=w96, "X Data.Path.a actual"=w91, "X Data.Path.V plan"=w56) -> (w40:T8)
    n182 = Unbundle By Name(w40) -> ("X Data.Path.Profile"=→"X Data.Path.Profile":T1, "Y Data.Path.Profile"=→"Y Data.Path. Profile":T1, "Timing"=→"Timing":T2, "X Data.State"=→"X Data.State":T3, "Y Data.State"=→"Y Data.State":T3, "X Data.Motor Params"=→"X Data.Motor Params":T7, "Y Data.Motor Params"=→"Y Data.Motor Params":T6, "X Data.Motion"=→"X Data.Motion":T5, "Y Data.Motion"=→"Y Data.Motion":T5, "X Data.Path.V plan"=w46:dbl[], "X Data.Path.V actual"=w45:dbl[], "Y Data.Path.V plan"=w43:dbl[], "Y Data.Path.V actual"=w42:dbl[], "X Data.Path.S actual"=→"X Displacement":dbl[], "X Data.Path.a actual"=→"X Acceleration":dbl[], "Y Data.Path.S actual"=→"Y Displacement":dbl[], "Y Data.Path.a actual"=→"Y Acceleration":dbl[], "X Data.Motor Params.Duty %"=→"X Duty%":dbl, "Y Data.Motor Params.Freq"=→"Y Freq":dbl, "X Data.SP.Speed"=w62:dbl, "X Data.Motion.Speed"=w61:dbl, "Y Data.SP.Speed"=w59:dbl, "Y Data.Motion.Speed"=w58:dbl, "X Data.Path.Decel Dist"=→"X Data.Path.Decel Dist":dbl, "Y Data.Path.Decel Dist"=→"Y Data.Path.Decel Dist":dbl)
    n183 = Build Cluster Array(w43, w42) -> (→"Y Velocity":cluster{"V actual":dbl[]}[])
    n184 = Build Cluster Array(w46, w45) -> (→"X Velocity":cluster{"V actual":dbl[]}[])
    n185 = Bundle("Speed"=w62, "Speed"=w61) -> (→"X PID":cluster{"Speed":dbl, "Speed":dbl})  [unwired: 1 in]
    n186 = Bundle("Speed"=w59, "Speed"=w58) -> (→"Y PID":cluster{"Speed":dbl, "Speed":dbl})  [unwired: 1 in]
    n187 = feedback #1(string[][] [] ("Initialised Array")) -> (w121:string[][])
    n188 = call "Compile Datalog Array sub_VI.vi"("XY Cluster"=w40, "Initialised Array"=w121) -> ("Data Array"=w122:string[][])  [unwired: 1 in]
    n189 = feedback-in #1(w122) -> ()
  }
